vi "BANDGAP DELTA POST TRIM - Read.vi"(8 "error in (no error)":errorcluster, 11 "Globals in":refnum<class "TSM Context Data Access.lvclass">) -> (0 "error out":errorcluster, 2 "BANDGAP DELTA POST TRIM":dbl[](array[numeric]), 3 "Globals out":refnum<class "TSM Context Data Access.lvclass">)   [LabVIEW 2019, in "TSM Context Data Access.lvclass"]
uses:
  TSM Context Data Access.lvclass
  TSM Context Data Access.lvclass/TSM Context Data Access.ctl
  <vilib>/NI_TestStand_SemiconductorModule/NI_TestStand_Semiconductor_Module.lvlibp
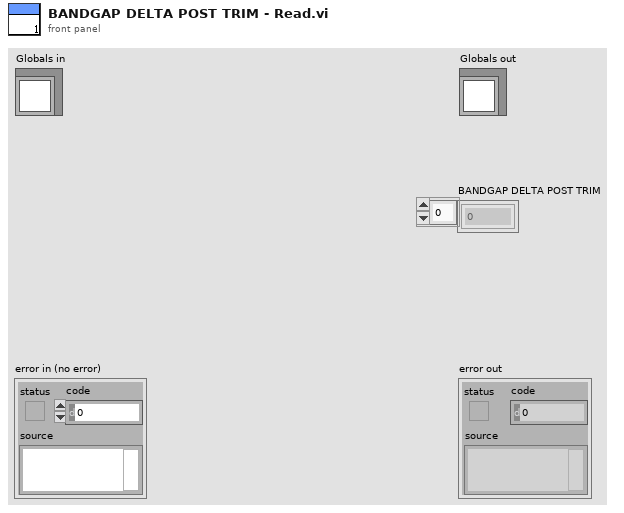
[diagram p1: front panel]
types:
  T1 = typedef "NI_TestStand_Semiconductor_Module.lvlibp/SemiconductorModuleContext.ctl" = refnum<k7>
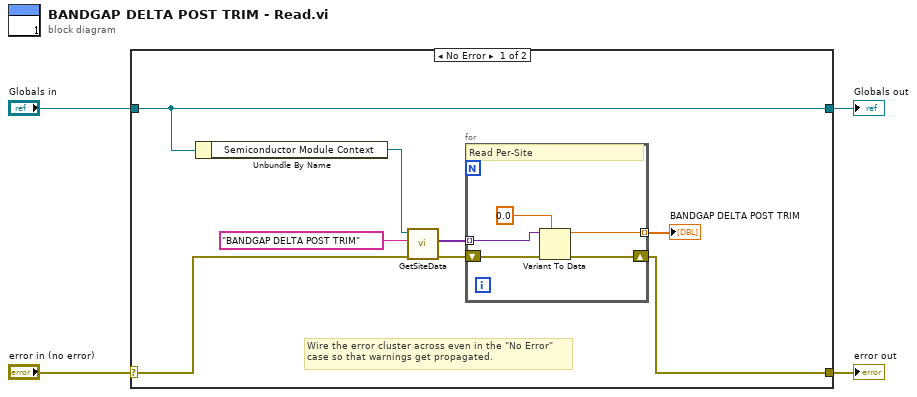
[diagram p0: block diagram]
diagram:
  n1 = case shown="No Error" "error in (no error)" {
    selector: "error in (no error)" -> [w8 w19]
    tunnel: [w7 w19] -> w3
    tunnel: [w6 w18] -> w1
    tunnel: "Globals in" -> [w6 w18]
    frame No Error {
      # "Wire the error cluster across even in the \"No Error\"\ncase so that warnings get propagated."
      n2 = Unbundle By Name(w6) -> ("Semiconductor Module Context"=w9:T1)
      n3 = call <vilib>:"GetSiteData.vi"("error in (no error)"=w8, "Data Id"="BANDGAP DELTA POST TRIM", "Semiconductor Module Context"=w9) -> ("error out"=w12:errorcluster, "Site Data"=w11:variant[])  [unwired: 6 in, 1 out]
      n4 = for {
        shift-right: [w16] -> w7
        shift-left: w12 -> [w17]
        tunnel: w11 -> [w15] mode=indexing
        tunnel: [w14] -> w5 mode=indexing
        # "Read Per-Site"
        n5 = Variant To Data(error in=w17, type=0.0, Variant=w15) -> (data=w14:dbl, error out=w16:errorcluster)
      }
      "BANDGAP DELTA POST TRIM" <- w5
    }
    frame Error {
    }
  }
  "error out" <- w3
  "Globals out" <- w1
